vi "Stim Timer.vi"(4 "Stim Timer Channel":T4, 5 "Timer Queue":refnum<queue>) -> (1 "Stim Channel":T3, 2 "Timer Status Channel":T2)   [LabVIEW 2019]
uses:
  <extravilib>/ChannelInstances/Messenger-t'Stim Timer Message.ctl'.lvlib
  Stim Interval Mode.ctl
  Protocol Interval.ctl
  Lee Lab/CP FES Walking 2018/Code/Working/LabVIEW/Controls/States/Stim Timer State.ctl
  Lee Lab/CP FES Walking 2018/Code/Working/LabVIEW/Controls/Messages/Stim Timer Message.ctl
  Timer Data.ctl
  Lee Lab/CP FES Walking 2018/Code/Working/LabVIEW/Controls/States/Stim State.ctl
  Lee Lab/CP FES Walking 2018/Code/Working/LabVIEW/Controls/Messages/Stim Message.ctl
  <extravilib>/ChannelInstances/Messenger-t'Stim Message.ctl'.lvlib
  CP FES State.ctl
  Messages/CP FES Message.ctl
  Lee Lab/CP FES Walking 2018/Code/Working/LabVIEW/Controls/States/Timer Status States.ctl
  Lee Lab/CP FES Walking 2018/Code/Working/LabVIEW/Controls/Messages/Timer Status Message.ctl
  <extravilib>/ChannelInstances/Messenger-t'Timer Status Message.ctl'.lvlib
  <extravilib>/ChannelInstances/Messenger-t'Stim Timer Message.ctl'/))Channel.ctl
  <extravilib>/ChannelInstances/Messenger-t'Stim Message.ctl'/))Channel.ctl
  <extravilib>/ChannelInstances/Messenger-t'Timer Status Message.ctl'/))Channel.ctl
panel:
  out "Stim Timer State":T1=enum."Off"
  out "Time to Next Interval":dbl[unit]
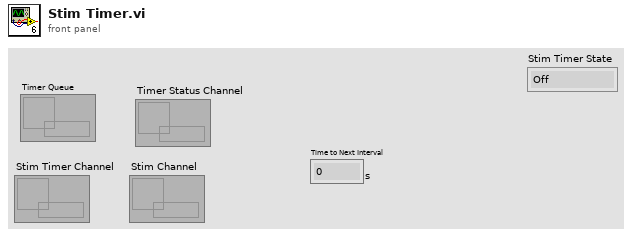
[diagram p1: front panel]
types:
  T1 = typedef "Stim Timer State.ctl" = enum16{"On", "Off", "Initialize", "Stop", "Alternating", "Pause", "Start Timer", "Reset Timer"}
  T2 = typedef "Messenger-t'Timer Status Message.ctl'.lvlib/))Channel.ctl" = refnum<queue>
  T3 = typedef "Messenger-t'Stim Message.ctl'.lvlib/))Channel.ctl" = refnum<queue>
  T4 = typedef "Messenger-t'Stim Timer Message.ctl'.lvlib/))Channel.ctl" = refnum<queue>
  T5 = typedef "Timer Data.ctl" = cluster{"Stim Timer State":T1, "Remaining session time":dbl[unit], "Curent interval duration":dbl[unit], "Time of last iteration":dbl[unit], "Time elapsed in current iteration":dbl[unit], "Current interval indicator":bool[], "Current interval number":u32, "Protocol":T6[], "Time to next interval":dbl[unit], "Mode":T7, "Alternating period":dbl[unit], "Alternating on or off":bool}
  T6 = typedef "Protocol Interval.ctl" = cluster{"Interval Type":enum16{"Walk", "Rest"}, "Duration":dbl[unit], " Mode":T7, "Alt Period":dbl[unit]}
  T7 = typedef "Stim Interval Mode.ctl" = enum32{"Stim", "No Stim", "Alternating"}
  T8 = typedef "Timer Status Message.ctl" = cluster{"Timer States":T9, "Data":variant}
  T9 = typedef "Timer Status States.ctl" = enum16{"Update"}
  T10 = typedef "Stim Timer Message.ctl" = cluster{"Stim Timer State":T1, "Data":variant}
  T11 = typedef "Stim Message.ctl" = cluster{"Stim State":T12, "Data":variant}
  T12 = typedef "Stim State.ctl" = enum16{"Initialize", "Open", "Idle", "Start Stim", "Update Params", "GPD Update", "Stop Stim", "Close", "Quit", "Clear Log"}
  T13 = typedef "CP FES Message.ctl" = cluster{"State":T14, "Data":variant}
  T14 = typedef "CP FES State.ctl" = enum16{"On", "Stop", "Idle", "Initialize", "Manual", "Stim On", "Stim Off", "Start Timer", "Pause", "Resume", "Reset"}
  T15 = typedef "Timer Data.ctl" = cluster{"Stim Timer State":T1, "Remaining session time":u32, "Curent interval duration":u32, "Time of last iteration":u32, "Time elapsed in current iteration":u32, "Current interval indicator":bool[], "Current interval number":u32, "Protocol":T16[], "Time to next interval":u32, "Mode":T7, "Alternating period":u32, "Alternating on or off":bool}
  T16 = typedef "Protocol Interval.ctl" = cluster{"Interval Type":enum16{"Walk", "Rest"}, "Duration":dbl, "Stim Mode":T7, "Alt Period":dbl}
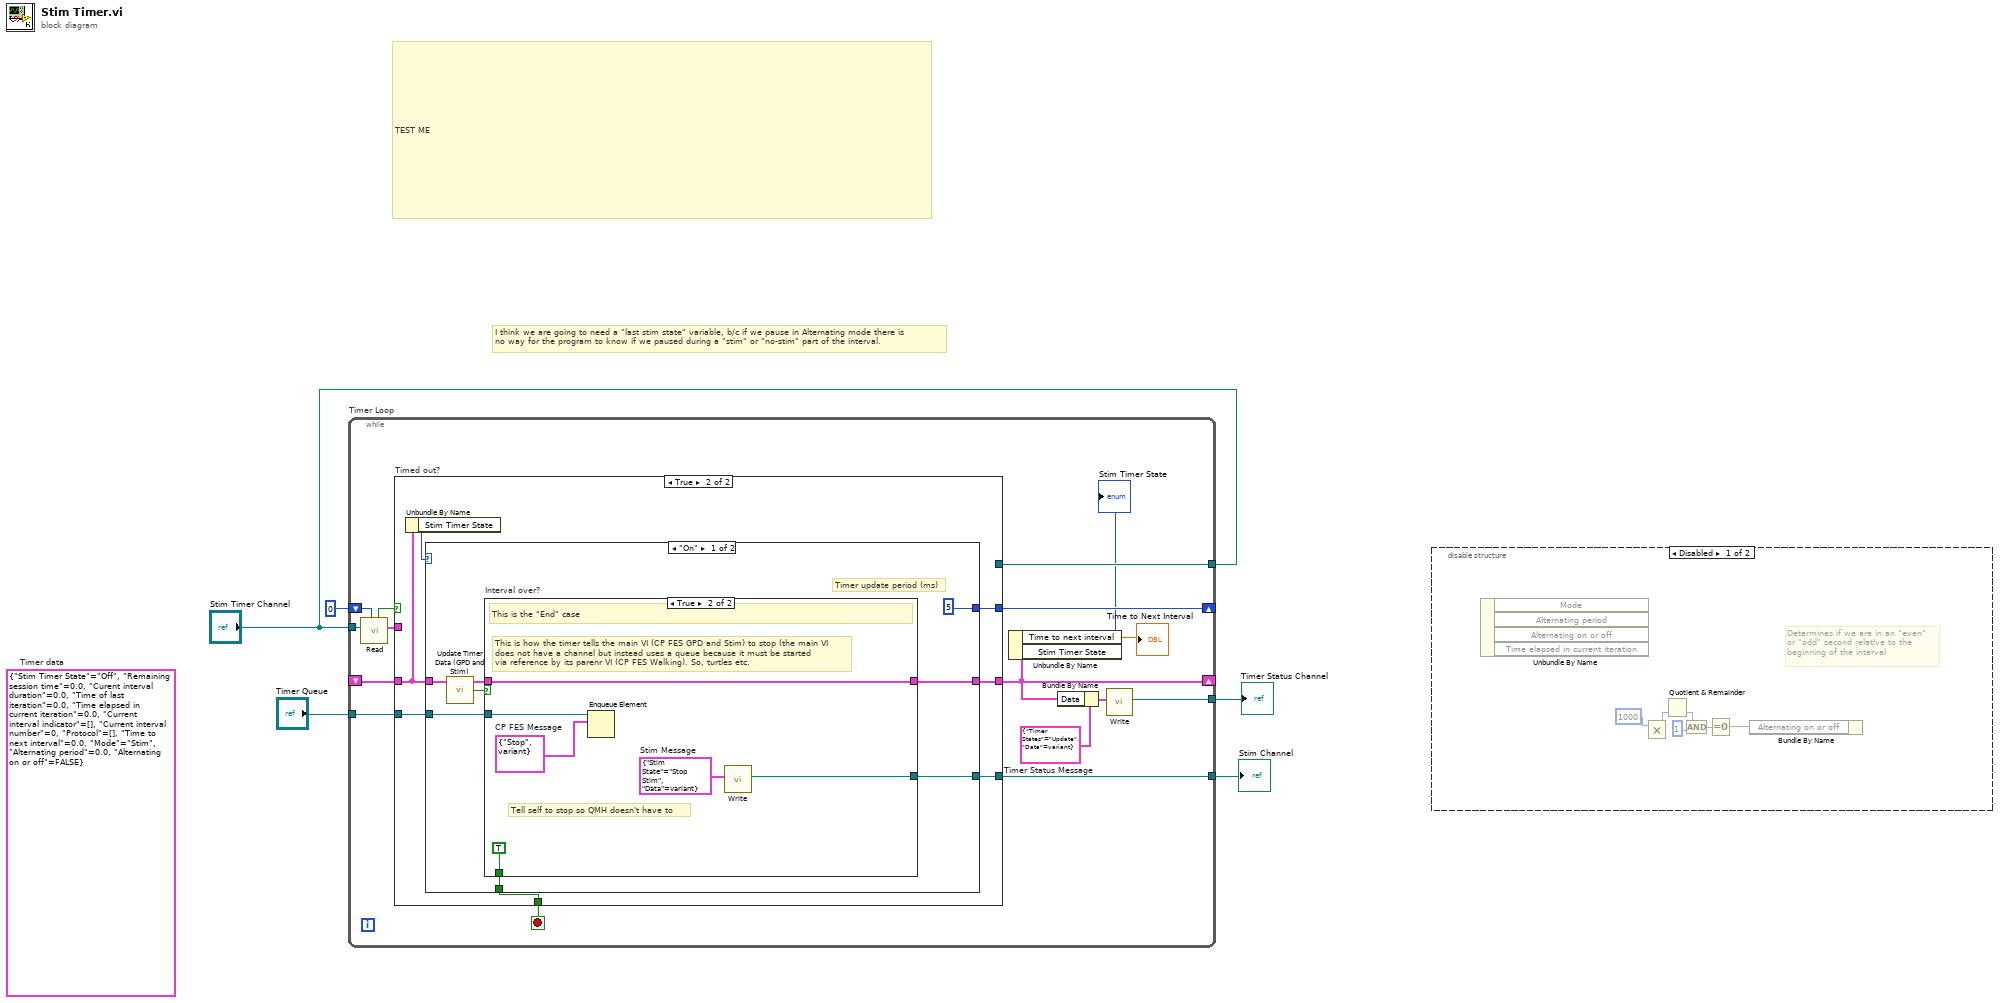
[diagram p0: block diagram]
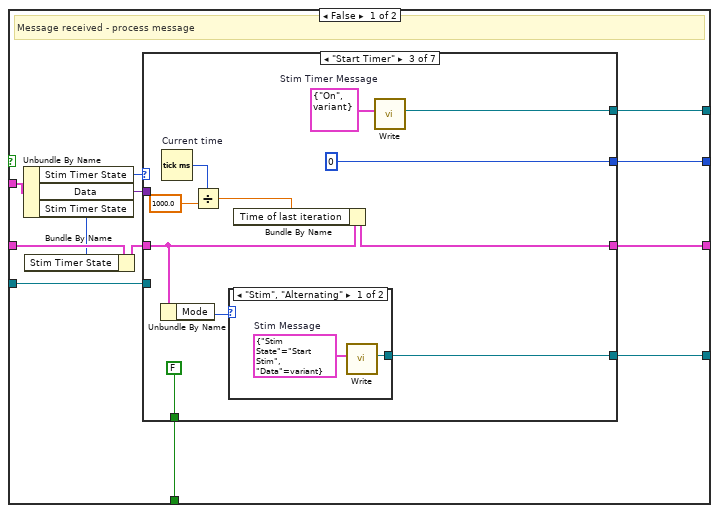
[diagram p3: hidden frame]
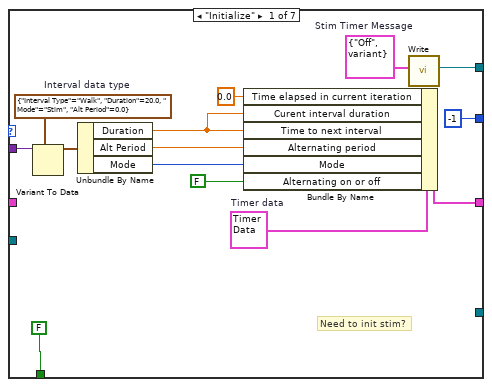
[diagram p4: hidden frame]
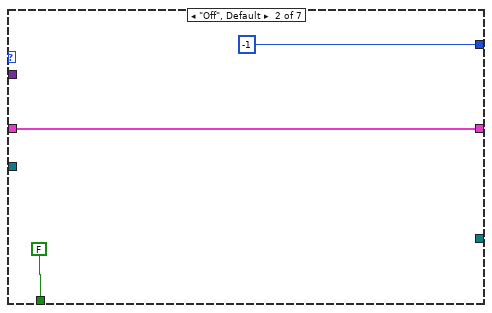
[diagram p5: hidden frame]
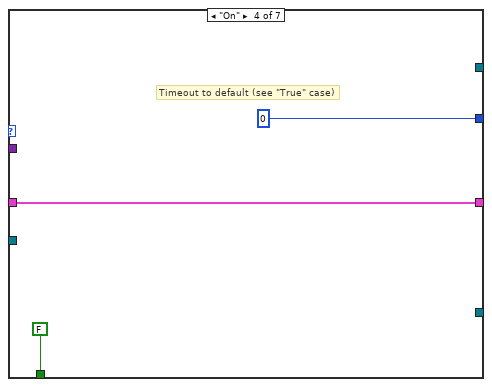
[diagram p7: hidden frame]
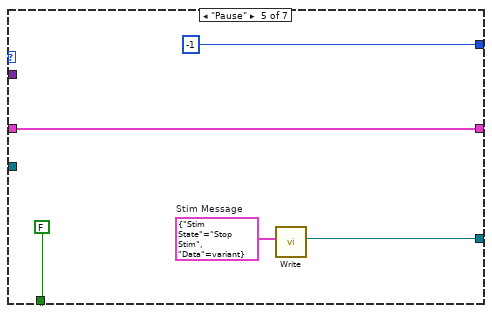
[diagram p8: hidden frame]
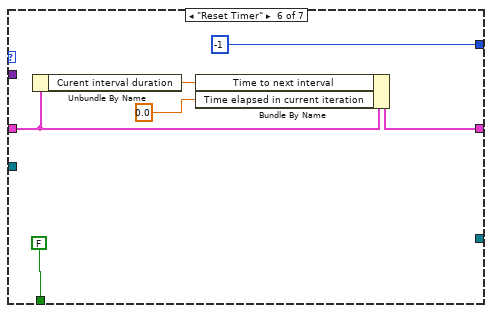
[diagram p9: hidden frame]
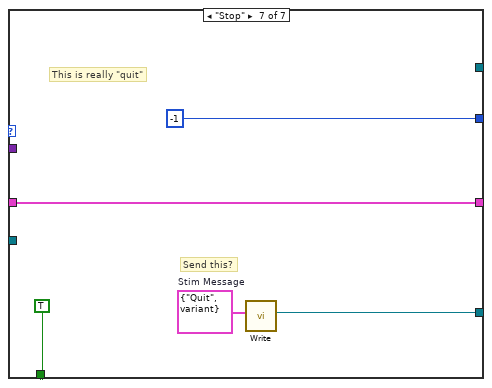
[diagram p10: hidden frame]
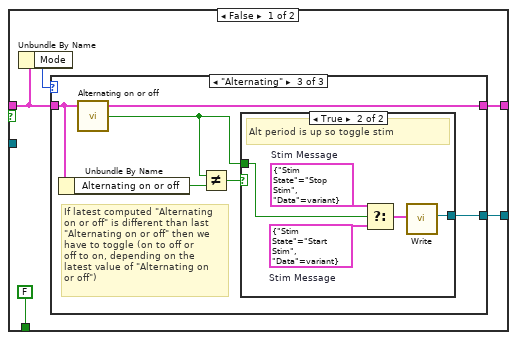
[diagram p11: hidden frame]
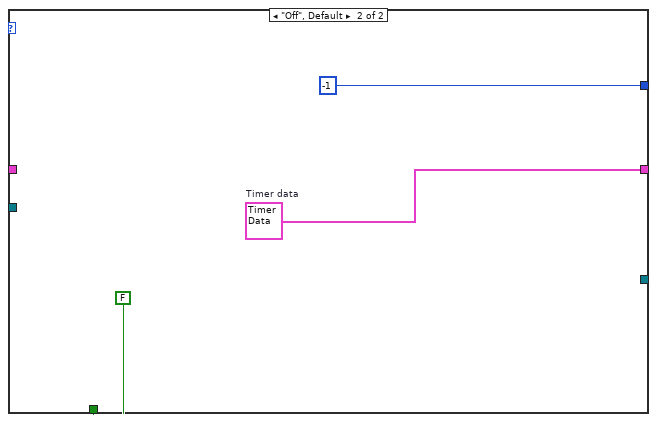
[diagram p15: hidden frame]
diagram:
  (unwired) T5 {"Stim Timer State"=enum."Off", "Remaining session time"=0.0, "Curent interval duration"=0.0, "Time of last iteration"=0.0, "Time elapsed in current iteration"=0.0, "Current interval indicator"=[], "Current interval number"=0, "Protocol"=[], "Time to next interval"=0.0, "Mode"=enum."Stim", "Alternating period"=0.0, "Alternating on or off"=FALSE}  # Timer data
  # "TEST ME"
  # "I think we are going to need a \"last stim state\" variable, b/c if we pause in Alternating mode there is\nno way for the program to know if we paused during a \"stim\" or \"no-stim\" part of the interval."
  n1 = while "Timer Loop" {
    tunnel: [w15] -> w4
    shift-right: [w14] -> _
    shift-left: _ -> [w19]
    tunnel: "Timer Queue" -> [w20]
    tunnel: "Stim Timer Channel" -> [w18]
    tunnel: "Stim Timer Channel" -> [w16]
    tunnel: [w11] -> w2
    shift-right: [w8] -> _
    shift-left: 0 ("milliseconds to wait") -> [w10]
    stop <- w21 stop-if-true
    w13 = T8 {"Timer States"=enum."Update", "Data"=variant}  # Timer Status Message
    n2 = call <extravilib>:"Read.vi"("timeout in ms (-1)"=w10, "channel"=w18) -> ("element"=w17:T10, "timedout?"=w9:bool)  [unwired: 6 in, 2 out]
    n3 = case "Timed out?" shown="True" w9 {
      tunnel: [w33 w88] -> w21
      tunnel: w20 -> [w32 w83]
      tunnel: w19 -> [w24 w86]
      tunnel: w17 -> [w28 _]
      tunnel: [w31 _] -> w16
      tunnel: [w30 w84] -> w15
      tunnel: [w29 w89] -> w14
      tunnel: [w25 w85] -> w8
      frame False {
        # "Message received - process message"
        n4 = Unbundle By Name(w28) -> ("Stim Timer State"=w27:T1, "Data"=w26:variant, "Stim Timer State"=w22:T1)
        n5 = Bundle By Name(cluster=w24, "Stim Timer State"=w22) -> (w23:T5)
        n6 = case shown="\"Start Timer\"" w27 {
          tunnel: [w44 w49 w60 w64 w70 w74 w81] -> w29
          tunnel: [FALSE FALSE FALSE FALSE FALSE FALSE TRUE] -> w33
          tunnel: [_ _ w58 _ w68 _ w79] -> w30
          tunnel: w32 -> [_ _ _ _ _ _ _]
          tunnel: w23 -> [_ w49 w55 w64 w70 w76 w81]
          tunnel: [w40 _ w56 _ _ _ _] -> w31
          tunnel: w26 -> [w38 _ _ _ _ _ _]
          tunnel: [-1 ("milliseconds to wait") -1 ("milliseconds to wait") 0 ("milliseconds to wait") 0 ("milliseconds to wait") -1 ("milliseconds to wait") -1 ("milliseconds to wait") -1 ("milliseconds to wait")] -> w25
          frame "Initialize" {
            w41 = T5 {"Stim Timer State"=enum."Off", "Remaining session time"=0.0, "Curent interval duration"=0.0, "Time of last iteration"=0.0, "Time elapsed in current iteration"=0.0, "Current interval indicator"=[], "Current interval number"=0, "Protocol"=[], "Time to next interval"=0.0, "Mode"=enum."No Stim", "Alternating period"=0.0, "Alternating on or off"=FALSE}  # Timer data
            w39 = T10 {"Stim Timer State"=enum."Off", "Data"=variant}  # Stim Timer Message
            w47 = T6 {"Interval Type"=enum."Walk", "Duration"=20.0, " Mode"=enum."Stim", "Alt Period"=0.0}  # Interval data type
            # "Need to init stim?"
            n7 = Variant To Data(type=w47, Variant=w38) -> (data=w46:T6)  [unwired: 1 in, 1 out]
            n8 = Unbundle By Name(w46) -> ("Duration"=w45:dbl[unit], "Alt Period"=w35:dbl[unit], "Mode"=w37:T7)
            n9 = Bundle By Name(cluster=w41, "Time elapsed in current iteration"=dbl[unit] 0.0, "Curent interval duration"=w45, "Time to next interval"=w45, "Alternating period"=w35, "Mode"=w37, "Alternating on or off"=FALSE) -> (w44:T5)
            n10 = call <extravilib>:"Write.vi"("element"=w39) -> ("channel"=w40:T4)  [unwired: 8 in, 2 out]
          }
          frame "Off", Default {
          }
          frame "Start Timer" {
            w57 = T10 {"Stim Timer State"=enum."On", "Data"=variant}  # Stim Timer Message
            n11 = Unbundle By Name(w55) -> ("Mode"=w59:T7)
            n12 = Tick Count (ms) "Current time"() -> (millisecond timer value=w53:u32)
            n13 = Divide(x=w53, y=dbl[unit] 1000.0) -> (x/y=w52:dbl[unit])
            n14 = case shown="\"Stim\", \"Alternating\"" w59 {
              tunnel: [w62 _] -> w58
              frame "Stim", "Alternating" {
                w63 = T11 {"Stim State"=enum."Start Stim", "Data"=variant}  # Stim Message
                n15 = call <extravilib>:"Write.vi"("element"=w63) -> ("channel"=w62:T3)  [unwired: 8 in, 2 out]
              }
              frame "No Stim", Default {
              }
            }
            n16 = Bundle By Name(cluster=w55, "Time of last iteration"=w52) -> (w60:T5)
            n17 = call <extravilib>:"Write.vi"("element"=w57) -> ("channel"=w56:T4)  [unwired: 8 in, 2 out]
          }
          frame "On" {
            # "Timeout to default (see \"True\" case)"
          }
          frame "Pause" {
            w69 = T11 {"Stim State"=enum."Stop Stim", "Data"=variant}  # Stim Message
            n18 = call <extravilib>:"Write.vi"("element"=w69) -> ("channel"=w68:T3)  [unwired: 8 in, 2 out]
          }
          frame "Reset Timer" {
            n19 = Unbundle By Name(w76) -> ("Curent interval duration"=w75:dbl[unit])
            n20 = Bundle By Name(cluster=w76, "Time to next interval"=w75, "Time elapsed in current iteration"=dbl[unit] 0.0) -> (w74:T5)
          }
          frame "Stop" {
            w80 = T11 {"Stim State"=enum."Quit", "Data"=variant}  # Stim Message
            # "This is really \"quit\""
            # "Send this?"
            n21 = call <extravilib>:"Write.vi"("element"=w80) -> ("channel"=w79:T3)  [unwired: 8 in, 2 out]
          }
        }
      }
      frame True {
        n22 = Unbundle By Name(w86) -> ("Stim Timer State"=w87:T1)
        n23 = case shown="\"On\"" w87 {
          tunnel: [w95 w124] -> w89
          tunnel: [w90 FALSE] -> w88
          tunnel: w86 -> [w91 _]
          tunnel: [5 ("milliseconds to wait") -1 ("milliseconds to wait")] -> w85
          tunnel: [w96 _] -> w84
          tunnel: w83 -> [w94 _]
          frame "On" {
            # "Timer update period (ms)"
            n24 = call "Update Timer Data (GPD and Stim).vi"("Timer Data In in"=w91) -> ("Interval Up?"=w92:bool, "Timer Data In out"=w93:T5)  [unwired: 3 in]
            n25 = case "Interval over?" shown="True" w92 {
              tunnel: [w99 w119] -> w95
              tunnel: [w102 w117] -> w96
              tunnel: w94 -> [_ w120]
              tunnel: w93 -> [w100 w119]
              tunnel: [FALSE TRUE] -> w90
              frame False {
                n26 = Unbundle By Name(w100) -> ("Mode"=w101:T7)
                n27 = case shown="\"Alternating\"" w101 {
                  tunnel: [_ _ w110] -> w102
                  tunnel: w100 -> [w103 w104 w108]
                  tunnel: [w103 w104 w105] -> w99
                  frame "Stim" {
                  }
                  frame "No Stim", Default {
                  }
                  frame "Alternating" {
                    # "If latest computed \"Alternating\non or off\" is different than last\n\"Alternating on or off\" then we \nhave to toggle (on to off or\noff to on, depending on the\nlatest value of \"Alternating on\nor off\")"
                    n28 = Unbundle By Name(w108) -> ("Alternating on or off"=w106:bool)
                    n29 = call "Alternating on or off"("Timer Data (GPD and Stim) in"=w108) -> ("Alternating on or off?"=w107:bool, "Timer Data (GPD and Stim) out"=w105:T5)  [unwired: 3 in]
                    n30 = Not Equal?(x=w107, y=w106) -> (x != y?=w109:bool)
                    n31 = case shown="True" w109 {
                      tunnel: w107 -> [_ w111]
                      tunnel: [_ w112] -> w110
                      frame False {
                        # "Alt period not up"
                      }
                      frame True {
                        w115 = T11 {"Stim State"=enum."Start Stim", "Data"=variant}  # Stim Message
                        w114 = T11 {"Stim State"=enum."Stop Stim", "Data"=variant}  # Stim Message
                        # "Alt period is up so toggle stim"
                        n32 = Select(t=w114, s=w111, f=w115) -> (s? t:f=w113:T11)
                        n33 = call <extravilib>:"Write.vi"("element"=w113) -> ("channel"=w112:T3)  [unwired: 8 in, 2 out]
                      }
                    }
                  }
                }
              }
              frame True {
                w118 = T11 {"Stim State"=enum."Stop Stim", "Data"=variant}  # Stim Message
                w121 = T13 {"State"=enum."Stop", "Data"=variant}  # CP FES Message
                # "This is how the timer tells the main VI (CP FES GPD and Stim) to stop (the main VI\ndoes not have a channel but instead uses a queue because it must be started \nvia reference by its parenr VI (CP FES Walking). So, turtles etc."
                # "Tell self to stop so QMH doesn't have to"
                # "This is the \"End\" case"
                n34 = Enqueue Element(queue=w120, element=w121) -> ()  [unwired: 2 in, 3 out]
                n35 = call <extravilib>:"Write.vi"("element"=w118) -> ("channel"=w117:T3)  [unwired: 8 in, 2 out]
              }
            }
          }
          frame "Off", Default {
            w124 = T5 {"Stim Timer State"=enum."Off", "Remaining session time"=0.0, "Curent interval duration"=0.0, "Time of last iteration"=0.0, "Time elapsed in current iteration"=0.0, "Current interval indicator"=[], "Current interval number"=0, "Protocol"=[], "Time to next interval"=0.0, "Mode"=enum."No Stim", "Alternating period"=0.0, "Alternating on or off"=FALSE}  # Timer data
          }
        }
      }
    }
    n36 = Unbundle By Name(w14) -> ("Time to next interval"=→"Time to Next Interval":dbl[unit], "Stim Timer State"=→"Stim Timer State":T1)
    n37 = Bundle By Name(cluster=w13, "Data"=w14) -> (w12:T8)
    n38 = call <extravilib>:"Write.vi"("element"=w12) -> ("channel"=w11:T2)  [unwired: 8 in, 2 out]
  }
  "Stim Channel" <- w4
  "Timer Status Channel" <- w2
  n39 = disable-structure shown="Disabled" {
    frame Disabled {
      # "Determines if we are in an \"even\"\nor \"odd\" second relative to the\nbeginning of the interval"
      n40 = Unbundle By Name() -> (w136:T15, "Mode"=w139, "Alternating period"=w138, "Alternating on or off"=w137, "Time elapsed in current iteration"=w135)
      n41 = Multiply(x=u32 1000 ("y")) -> (y=w126:u32, x*y=w131:u32)
      n42 = Quotient & Remainder(y=w131) -> (x=w125:u32, floor(x/y)=w132:u32)  [unwired: 1 out]
      n43 = And(x=w132, y=u32 1) -> (x .and. y?=w133:u32)
      n44 = Equal To 0?(x=w133) -> (x = 0?=w129:bool)
      n45 = Bundle By Name("Alternating on or off"=w129) -> (w128:cluster{}, w130:cluster{})
    }
    frame Enabled {
    }
  }
